vi "UpdatePupilTrackingData.vi"(2 "Circle fit parameters in":T1, 3 "Fitted Circle":T2) -> (0 "Circle fit parameters out":T1, 1 "Rectangle":i32[](array[numeric]))   [LabVIEW 2013]
doc: "Updates Circle Fit parameters with the latest results from the circle fitting. Also outputs the coordinates for the fitted circle in the original image."
uses:
  TrackingParameters.ctl
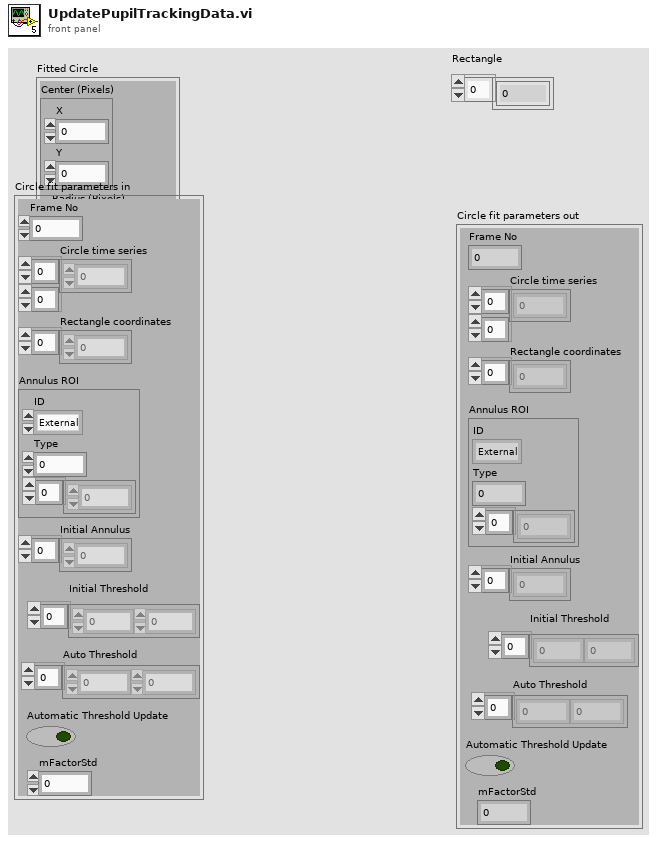
[diagram p1: front panel]
types:
  T1 = typedef "TrackingParameters.ctl" = cluster{"Frame No":i32, "Circle time series":dbl[][], "Rectangle coordinates":i32[], "Annulus ROI":cluster{"ID":enum32{"External", "Internal"}, "Type":u32, i32[]}, "Initial Annulus":i32[], "Auto Threshold":sgl[], "Automatic Threshold Update":bool, "Initial Threshold":sgl[], "mFactorStd":dbl}
  T2 = cluster{"Center (Pixels)":cluster{"X":sgl, "Y":sgl}, "Radius (Pixels)":dbl, "Center (Real-World)":cluster{"X":sgl, "Y":sgl}, "Radius (Real-World)":dbl, "Roundness (Real-World)":dbl, "Average Strength":dbl, "Average SNR (dB)":dbl}
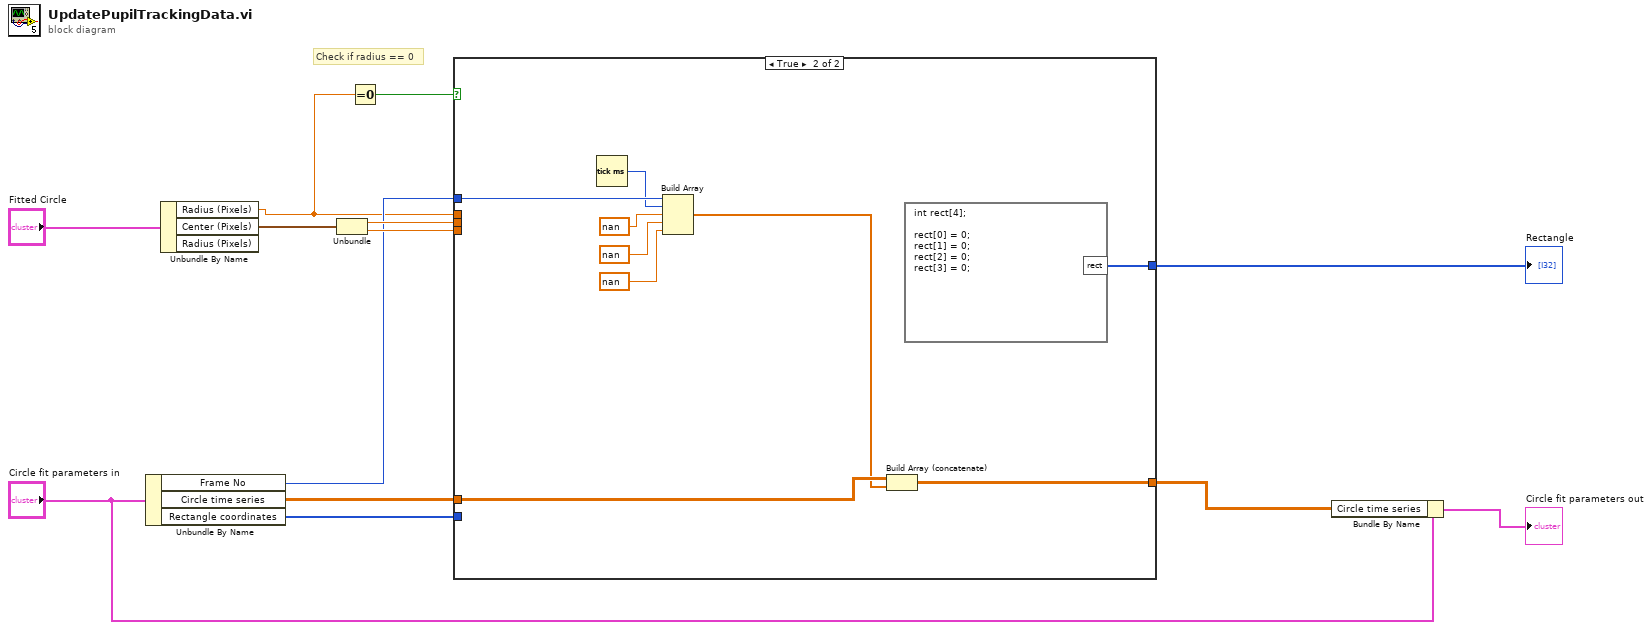
[diagram p0: block diagram]
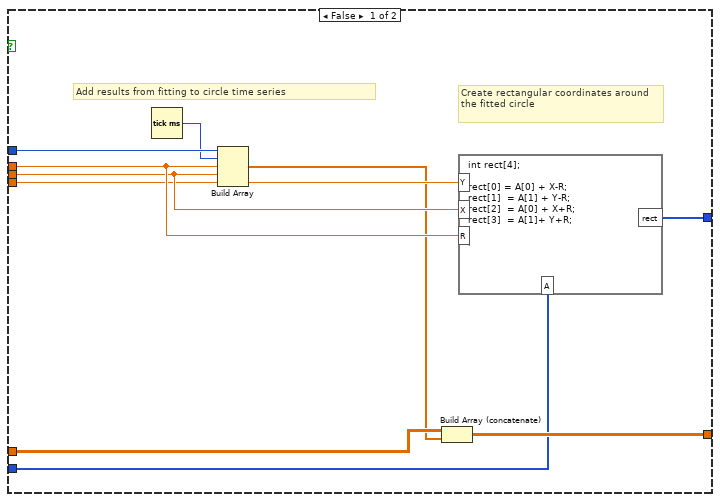
[diagram p2: hidden frame]
diagram:
  # "Check if radius == 0"
  n1 = Unbundle By Name("Circle fit parameters in") -> ("Frame No"=w5:i32, "Circle time series"=w6:dbl[][], "Rectangle coordinates"=w7:i32[])
  n2 = Unbundle By Name("Fitted Circle") -> ("Radius (Pixels)"=w1:dbl, "Center (Pixels)"=w12:cluster{"X":sgl, "Y":sgl})  [unwired: 1 out]
  n3 = Unbundle(w12) -> ("X"=w10:sgl, "Y"=w9:sgl)
  n4 = Equal To 0?(x=w1) -> (x = 0?=w13:bool)
  n5 = case shown="True" w13 {
    tunnel: w6 -> [w22 w28]
    tunnel: [w23 w29] -> w3
    tunnel: w1 -> [w18 _]
    tunnel: w10 -> [w17 _]
    tunnel: w9 -> [w16 _]
    tunnel: w5 -> [w21 w26]
    tunnel: [w19 w24] -> w8
    tunnel: w7 -> [w14 _]
    frame False {
      # "Create rectangular coordinates around the fitted circle"
      # "Add results from fitting to circle time series"
      n6 = Tick Count (ms)() -> (millisecond timer value=w20:u32)
      n7 = Build Array(w21, w20, w18, w17, w16) -> (w15:dbl[])
      n8 = Build Array (concatenate)(w22, w15) -> (w23:dbl[][])
      n9 = formula code="int rect[4];\n\nrect[0] = A[0] + X-R;\nrect[1]  = A[1] + Y-R;\nrect[2]  = A[0] + X+R;\nrect[3]  = A[1]+ Y+R;\n\n;"("X"=w17, "Y"=w16, "R"=w18, "A"=w14) -> ("rect"=w19:i32[])
    }
    frame True {
      n10 = Tick Count (ms)() -> (millisecond timer value=w25:u32)
      n11 = Build Array(w26, w25, nan, nan, nan) -> (w27:dbl[])
      n12 = Build Array (concatenate)(w28, w27) -> (w29:dbl[][])
      n13 = formula code="int rect[4];\n\nrect[0] = 0;\nrect[1] = 0;\nrect[2] = 0;\nrect[3] = 0;"() -> ("rect"=w24:i32[])
    }
  }
  "Rectangle" <- w8
  n14 = Bundle By Name(cluster="Circle fit parameters in", "Circle time series"=w3) -> (→"Circle fit parameters out":T1)
